vi "ID Finder Motor.vi"(0 "cluster":T3 {"data[0]"."payload" format="%x"; "data[0]"."timestamp" format="%<%.7X\n%x>T"; "data[0]"."type" items=["CAN Data"=0, "CAN Remote"=1, "CAN Bus Error"=2, "CAN 2.0 Data"=8, "CAN FD Data"=16, "CAN FD+BRS Data"=24, "J1939 Data"=192, "Delay"=224, "Log Trigger"=225, "Start Trigger"=226]; "data[0]"."identifier" format="%x"; "data[1]"."payload" format="%x"; "data[1]"."timestamp" format="%<%.7X\n%x>T"; "data[1]"."type" items=["CAN Data"=0, "CAN Remote"=1, "CAN Bus Error"=2, "CAN 2.0 Data"=8, "CAN FD Data"=16, "CAN FD+BRS Data"=24, "J1939 Data"=192, "Delay"=224, "Log Trigger"=225, "Start Trigger"=226]; "data[1]"."identifier" format="%x"; "data[2]"."payload" format="%x"; "data[2]"."timestamp" format="%<%.7X\n%x>T"; "data[2]"."type" items=["CAN Data"=0, "CAN Remote"=1, "CAN Bus Error"=2, "CAN 2.0 Data"=8, "CAN FD Data"=16, "CAN FD+BRS Data"=24, "J1939 Data"=192, "Delay"=224, "Log Trigger"=225, "Start Trigger"=226]; "data[2]"."identifier" format="%x"; "data[3]"."payload" format="%x"; "data[3]"."timestamp" format="%<%.7X\n%x>T"; "data[3]"."type" items=["CAN Data"=0, "CAN Remote"=1, "CAN Bus Error"=2, "CAN 2.0 Data"=8, "CAN FD Data"=16, "CAN FD+BRS Data"=24, "J1939 Data"=192, "Delay"=224, "Log Trigger"=225, "Start Trigger"=226]; "data[3]"."identifier" format="%x"; "data[4]"."payload" format="%x"; "data[4]"."timestamp" format="%<%.7X\n%x>T"; "data[4]"."type" items=["CAN Data"=0, "CAN Remote"=1, "CAN Bus Error"=2, "CAN 2.0 Data"=8, "CAN FD Data"=16, "CAN FD+BRS Data"=24, "J1939 Data"=192, "Delay"=224, "Log Trigger"=225, "Start Trigger"=226]; "data[4]"."identifier" format="%x"; "data[5]"."payload" format="%x"; "data[5]"."timestamp" format="%<%.7X\n%x>T"; "data[5]"."type" items=["CAN Data"=0, "CAN Remote"=1, "CAN Bus Error"=2, "CAN 2.0 Data"=8, "CAN FD Data"=16, "CAN FD+BRS Data"=24, "J1939 Data"=192, "Delay"=224, "Log Trigger"=225, "Start Trigger"=226]; "data[5]"."identifier" format="%x"; "data[6]"."payload" format="%x"; "data[6]"."timestamp" format="%<%.7X\n%x>T"; "data[6]"."type" items=["CAN Data"=0, "CAN Remote"=1, "CAN Bus Error"=2, "CAN 2.0 Data"=8, "CAN FD Data"=16, "CAN FD+BRS Data"=24, "J1939 Data"=192, "Delay"=224, "Log Trigger"=225, "Start Trigger"=226]; "data[6]"."identifier" format="%x"; "data[7]"."payload" format="%x"; "data[7]"."timestamp" format="%<%.7X\n%x>T"; "data[7]"."type" items=["CAN Data"=0, "CAN Remote"=1, "CAN Bus Error"=2, "CAN 2.0 Data"=8, "CAN FD Data"=16, "CAN FD+BRS Data"=24, "J1939 Data"=192, "Delay"=224, "Log Trigger"=225, "Start Trigger"=226]; "data[7]"."identifier" format="%x"; "data[8]"."payload" format="%x"; "data[8]"."timestamp" format="%<%.7X\n%x>T"; "data[8]"."type" items=["CAN Data"=0, "CAN Remote"=1, "CAN Bus Error"=2, "CAN 2.0 Data"=8, "CAN FD Data"=16, "CAN FD+BRS Data"=24, "J1939 Data"=192, "Delay"=224, "Log Trigger"=225, "Start Trigger"=226]; "data[8]"."identifier" format="%x"}, 1 "ID ESPERADO STRING":string) -> (3 "Data String 8":string, 4 "Data String 3":string, 5 "Data String 2":string, 6 "ID String":string, 7 "Data String 4":string, 8 "Data String 7":string, 10 "Data String 10":string, 11 "Data String 6":string, 12 "Identifier":u32 format="%x", 13 "Data Type":T1 items=["CAN Data"=0, "CAN Remote"=1, "CAN Bus Error"=2, "CAN 2.0 Data"=8, "CAN FD Data"=16, "CAN FD+BRS Data"=24, "J1939 Data"=192, "Delay"=224, "Log Trigger"=225, "Start Trigger"=226], 14 "Timestamp":timestamp, 15 "Payload":u8[](array[numeric]) format="%x", 17 "Data String 5":string, 18 "Data String 9":string, 19 "Data String":string)   [LabVIEW 2023]
uses:
  <vilib>/xnet/xnet.llb/XNET Frame CAN.ctl
  <vilib>/xnet/xnet.llb/XNET Frame Type CAN.ctl
  C:/Elatch-Bench-Test/VIs 64 bits/Users/k90011005/Desktop/Practicas/C#/String-Hexa/bin/Debug/String-Hexa.dll
  VIs 64 bits/Users/k90011005/Desktop/Practicas/C#/String-Hexa/bin/Debug/String-Hexa.dll
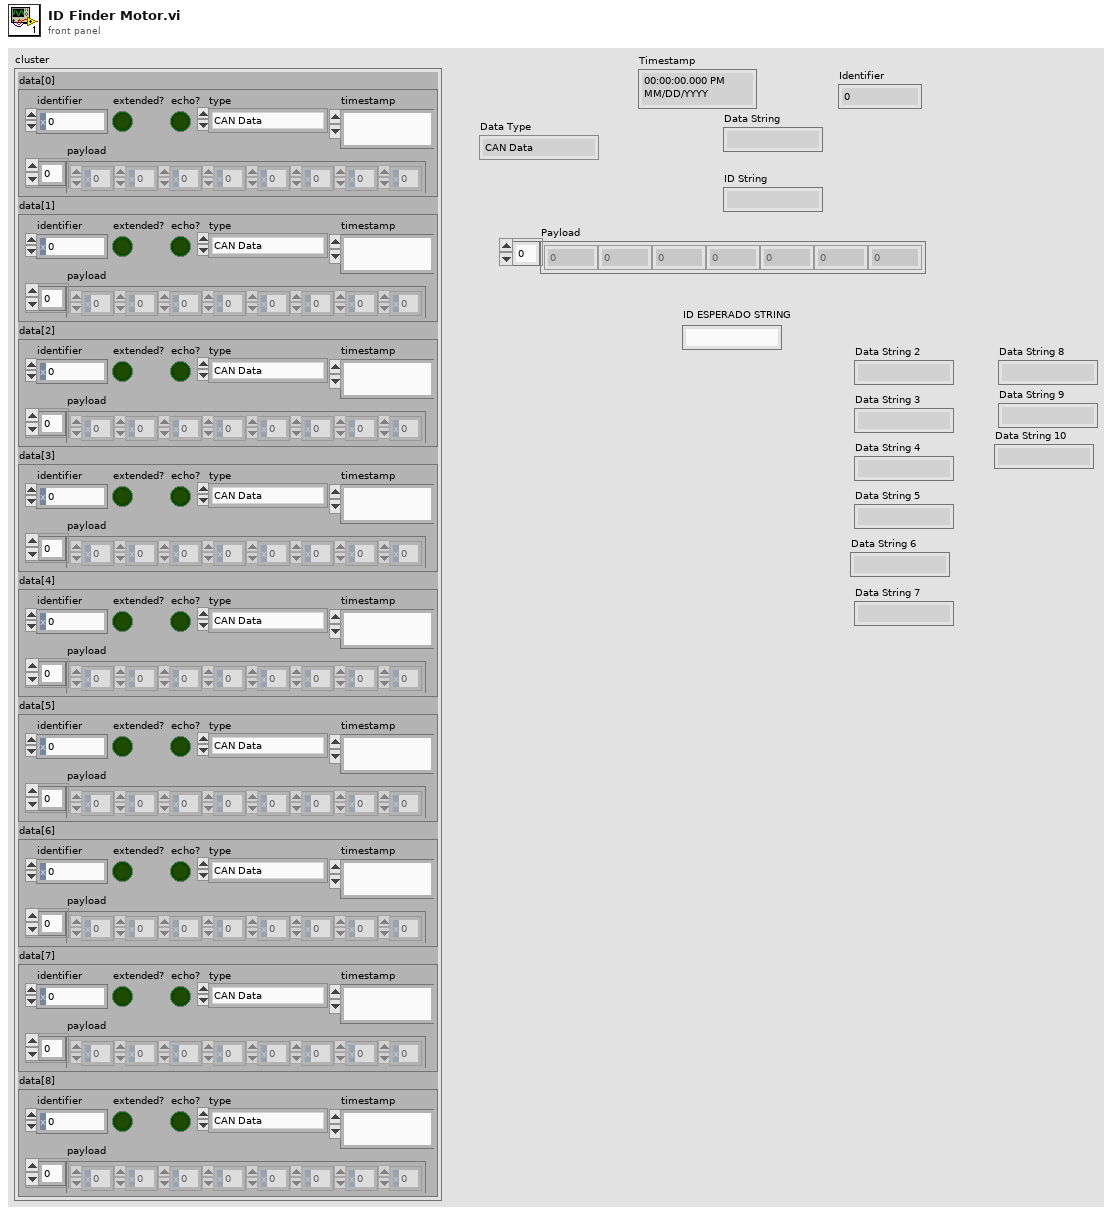
[diagram p1: front panel]
types:
  T1 = typedef "XNET Frame Type CAN.ctl" = u8
  T2 = typedef "XNET Frame CAN.ctl" = cluster{"timestamp":timestamp, "payload":u8[], "identifier":u32, "type":T1, "extended?":bool, "echo?":bool}
  T3 = cluster{"data[0]":T2, "data[1]":T2, "data[2]":T2, "data[3]":T2, "data[4]":T2, "data[5]":T2, "data[6]":T2, "data[7]":T2, "data[8]":T2}
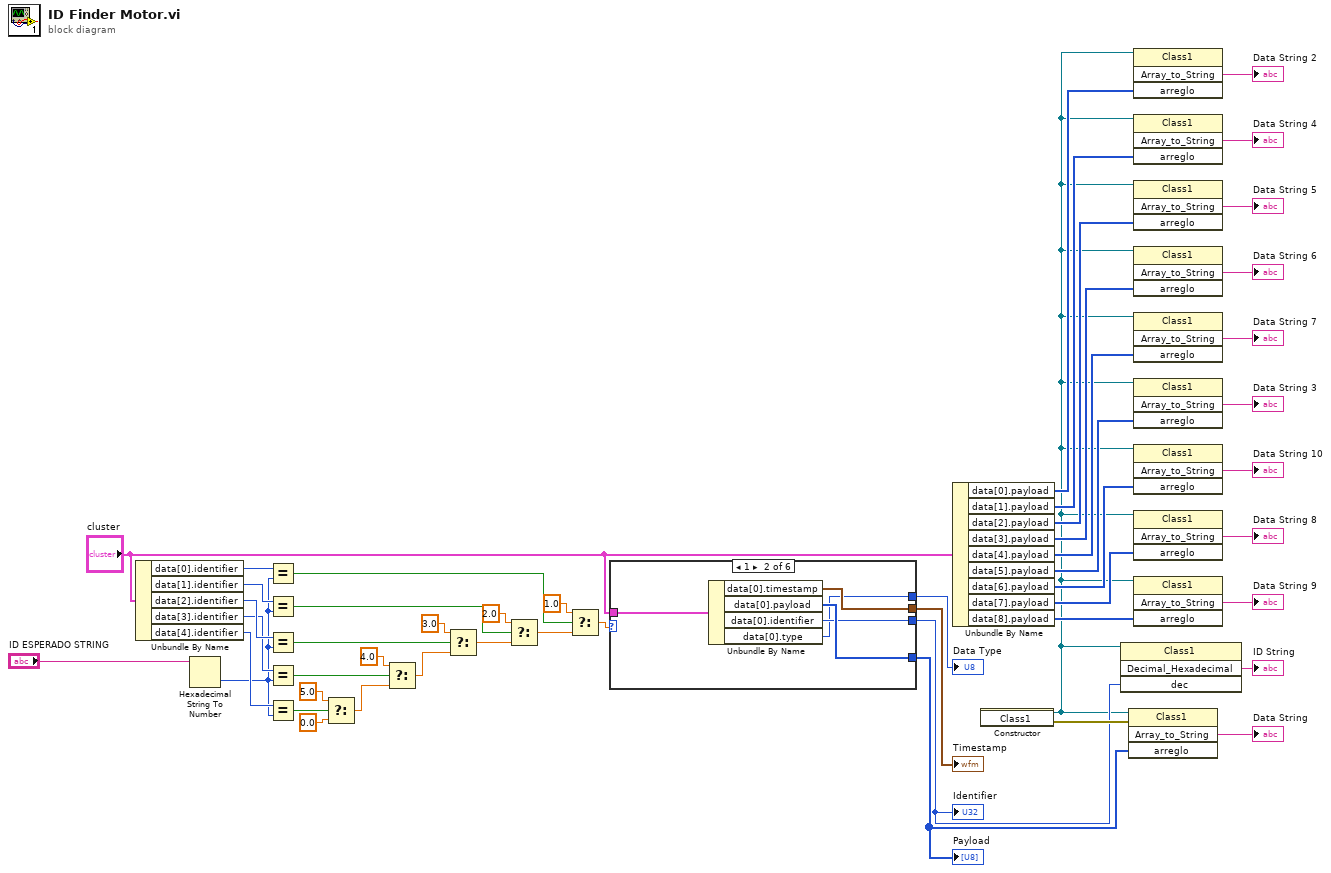
[diagram p0: block diagram]
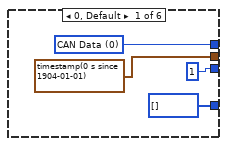
[diagram p2: hidden frame]
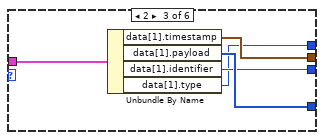
[diagram p3: hidden frame]
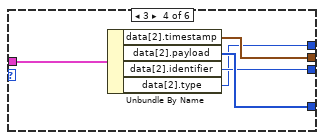
[diagram p4: hidden frame]
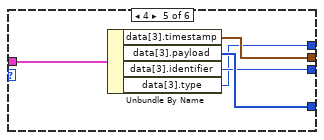
[diagram p5: hidden frame]
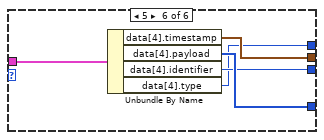
[diagram p6: hidden frame]
diagram:
  n1 = Unbundle By Name("cluster") -> ("data[0].identifier"=w50:u32, "data[1].identifier"=w46:u32, "data[2].identifier"=w45:u32, "data[3].identifier"=w44:u32, "data[4].identifier"=w43:u32)
  n2 = Hexadecimal String To Number(string="ID ESPERADO STRING") -> (number=w21:u32)  [unwired: 2 in, 1 out]
  n3 = Equal?(x=w50, y=w21) -> (x = y?=w49:bool)
  n4 = Equal?(x=w46, y=w21) -> (x = y?=w38:bool)
  n5 = Equal?(x=w45, y=w21) -> (x = y?=w37:bool)
  n6 = Equal?(x=w44, y=w21) -> (x = y?=w36:bool)
  n7 = Equal?(x=w43, y=w21) -> (x = y?=w35:bool)
  n8 = Select(t=5.0, s=w35, f=0.0) -> (s? t:f=w39:dbl)
  n9 = Select(t=4.0, s=w36, f=w39) -> (s? t:f=w40:dbl)
  n10 = Select(t=3.0, s=w37, f=w40) -> (s? t:f=w41:dbl)
  n11 = Select(t=2.0, s=w38, f=w41) -> (s? t:f=w42:dbl)
  n12 = Select(t=1.0, s=w49, f=w42) -> (s? t:f=w47:dbl)
  n13 = case shown="1" w47 {
    tunnel: "cluster" -> [_ w59 w64 w69 w74 w79]
    tunnel: [timestamp(0 s since 1904-01-01) ("timestamp") w58 w63 w68 w73 w78] -> w29
    tunnel: [u8[] [] ("payload") w57 w62 w67 w72 w77] -> w26
    tunnel: [u32 1 ("identifier") w56 w61 w66 w71 w76] -> w24
    tunnel: [w51 w55 w60 w65 w70 w75] -> w28
    frame 0, Default {
      w51 = T1 0 items=["CAN Data"=0, "CAN Remote"=1, "CAN Bus Error"=2, "CAN 2.0 Data"=8, "CAN FD Data"=16, "CAN FD+BRS Data"=24, "J1939 Data"=192, "Delay"=224, "Log Trigger"=225, "Start Trigger"=226] ("type")
    }
    frame 1 {
      n14 = Unbundle By Name(w59) -> ("data[0].timestamp"=w58:timestamp, "data[0].payload"=w57:u8[], "data[0].identifier"=w56:u32, "data[0].type"=w55:T1)
    }
    frame 2 {
      n15 = Unbundle By Name(w64) -> ("data[1].timestamp"=w63:timestamp, "data[1].payload"=w62:u8[], "data[1].identifier"=w61:u32, "data[1].type"=w60:T1)
    }
    frame 3 {
      n16 = Unbundle By Name(w69) -> ("data[2].timestamp"=w68:timestamp, "data[2].payload"=w67:u8[], "data[2].identifier"=w66:u32, "data[2].type"=w65:T1)
    }
    frame 4 {
      n17 = Unbundle By Name(w74) -> ("data[3].timestamp"=w73:timestamp, "data[3].payload"=w72:u8[], "data[3].identifier"=w71:u32, "data[3].type"=w70:T1)
    }
    frame 5 {
      n18 = Unbundle By Name(w79) -> ("data[4].timestamp"=w78:timestamp, "data[4].payload"=w77:u8[], "data[4].identifier"=w76:u32, "data[4].type"=w75:T1)
    }
  }
  "Timestamp" <- w29
  "Payload" <- w26
  "Identifier" <- w24
  "Data Type" <- w28
  n19 = Unbundle By Name("cluster") -> ("data[0].payload"=w19:u8[], "data[1].payload"=w18:u8[], "data[2].payload"=w17:u8[], "data[3].payload"=w16:u8[], "data[4].payload"=w15:u8[], "data[5].payload"=w14:u8[], "data[6].payload"=w7:u8[], "data[7].payload"=w6:u8[], "data[8].payload"=w5:u8[])
  n20 = constructor class="Class1"() -> (reference out=w1:refnum<k24>, error out=w27:errorcluster)  [unwired: 3 in, 1 out]
  n21 = invoke class="Class1" method="Decimal_Hexadecimal"(reference=w1, "dec"=w24) -> ("Decimal_Hexadecimal"=→"ID String":string)  [unwired: 2 in, 3 out]
  n22 = invoke class="Class1" method="Array_to_String"(reference=w1, error in=w27, "arreglo"=w26) -> ("Array_to_String"=→"Data String":string)  [unwired: 1 in, 3 out]
  n23 = invoke class="Class1" method="Array_to_String"(reference=w1, "arreglo"=w19) -> ("Array_to_String"=→"Data String 2":string)  [unwired: 2 in, 3 out]
  n24 = invoke class="Class1" method="Array_to_String"(reference=w1, "arreglo"=w18) -> ("Array_to_String"=→"Data String 4":string)  [unwired: 2 in, 3 out]
  n25 = invoke class="Class1" method="Array_to_String"(reference=w1, "arreglo"=w17) -> ("Array_to_String"=→"Data String 5":string)  [unwired: 2 in, 3 out]
  n26 = invoke class="Class1" method="Array_to_String"(reference=w1, "arreglo"=w16) -> ("Array_to_String"=→"Data String 6":string)  [unwired: 2 in, 3 out]
  n27 = invoke class="Class1" method="Array_to_String"(reference=w1, "arreglo"=w15) -> ("Array_to_String"=→"Data String 7":string)  [unwired: 2 in, 3 out]
  n28 = invoke class="Class1" method="Array_to_String"(reference=w1, "arreglo"=w14) -> ("Array_to_String"=→"Data String 3":string)  [unwired: 2 in, 3 out]
  n29 = invoke class="Class1" method="Array_to_String"(reference=w1, "arreglo"=w7) -> ("Array_to_String"=→"Data String 10":string)  [unwired: 2 in, 3 out]
  n30 = invoke class="Class1" method="Array_to_String"(reference=w1, "arreglo"=w6) -> ("Array_to_String"=→"Data String 8":string)  [unwired: 2 in, 3 out]
  n31 = invoke class="Class1" method="Array_to_String"(reference=w1, "arreglo"=w5) -> ("Array_to_String"=→"Data String 9":string)  [unwired: 2 in, 3 out]
